vi "Function_Find Circle #2.vi"(7 "功能":enum16{"半徑", "毛邊"}(ring), 8 "Error in":errorcluster, 9 "CoordSys In":T2 {"Measurement System"."Axis Reference" items=["Direct", "Indirect"]; "Measurement System"."Angle (deg)" format="%.2f"; "Measurement System"."Origin"."Y" format="%.2f"; "Measurement System"."Origin"."X" format="%.2f"; "Reference System"."Axis Reference" items=["Direct", "Indirect"]; "Reference System"."Angle (deg)" format="%.2f"; "Reference System"."Origin"."Y" format="%.2f"; "Reference System"."Origin"."X" format="%.2f"}, 10 "Data Cluster In":cluster{"Name":string, "Variant In":variant}, 11 "Image Src":T4) -> (0 "Error Out":errorcluster, 1 "Max & min":T1 {"Min Position"."Y" format="%.2f"; "Min Position"."X" format="%.2f"; "Max Position"."Y" format="%.2f"; "Max Position"."X" format="%.2f"}, 2 "Result(Circ)":cluster{"Name":string, "NG?":bool, "Score":dbl}, 3 "Result":T3 {"Center"."Y" format="%.2f"; "Center"."X" format="%.2f"}, 4 "Time":u32)   [LabVIEW 2013]
uses:
  <vilib>/vision/Image Controls.llb/IMAQ Image.ctl
  Control/Control Find Circle #2.ctl
  <vilib>/vision/Measure.llb/Edge Options.ctl
  <vilib>/vision/Measure.llb/Edge Polarity.ctl
  <vilib>/vision/NI_Vision_Development_Module.lvlib
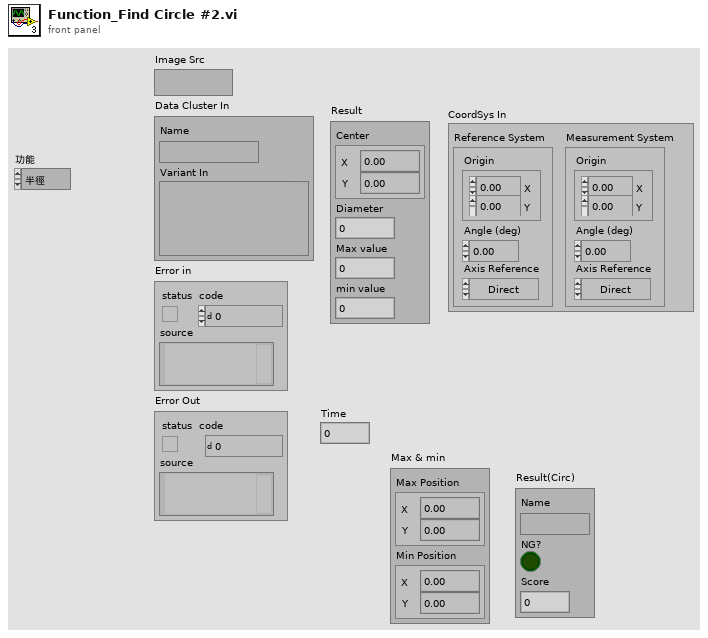
[diagram p1: front panel]
types:
  T1 = cluster{"Max Position":cluster{"X":sgl, "Y":sgl}, "Min Position":cluster{"X":sgl, "Y":sgl}}
  T2 = typedef "IMAQ Coordinate System" = cluster{"Reference System":cluster{"Origin":cluster{"X":sgl, "Y":sgl}, "Angle (deg)":sgl, "Axis Reference":u32}, "Measurement System":cluster{"Origin":cluster{"X":sgl, "Y":sgl}, "Angle (deg)":sgl, "Axis Reference":u32}}
  T3 = cluster{"Center":cluster{"X":sgl, "Y":sgl}, "Diameter":dbl, "Max value":sgl, "min value":sgl}
  T4 = typedef "IMAQ Image.ctl" = refnum<image>
  T5 = typedef "Control Find Circle #2.ctl" = cluster{"ROI Descriptor":cluster{"Global Rectangle":i32[], "Contours":cluster{"ID":enum32{"External", "Internal"}, "Type":u32, "Coordinates":i32[]}[]}, "Edge Options":cluster{"Edge Options":T6, "Step Size":dbl, "Scan Direction":u16, "Auto":bool, "SD":dbl}, "條件":cluster{"半徑最大值":dbl, "半徑最小值":dbl}}
  T6 = typedef "Edge Options.ctl" = cluster{"Edge Polarity":T7, "Kernel Size":u32, "Width":u32, "Minimum Edge Strength":sgl, "Interpolation Type":enum32{"Zero Order", "Bilinear", "Quadratic", "Cubic", "Bilinear Fixed"}, "Data Processing Method":enum32{"Average", "Median"}}
  T7 = typedef "Edge Polarity.ctl" = u32
  T8 = cluster{"Center":cluster{"X":sgl, "Y":sgl}, "Radius":dbl, "Max value":sgl, "min value":sgl}
  T9 = cluster{"Global Rectangle":i32[], "Contours":cluster{"ID":enum32{"External", "Internal"}, "Type":u32, "Coordinates":i32[]}[]}
  T10 = cluster{"Origin":cluster{"X":sgl, "Y":sgl}, "Angle (deg)":sgl, "Axis Reference":u32}
  T11 = typedef "ROI Descriptor" = cluster{"Global Rectangle":i32[], "Contours":cluster{"ID":enum32{"External", "Internal"}, "Type":u32, "Coordinates":i32[]}[]}
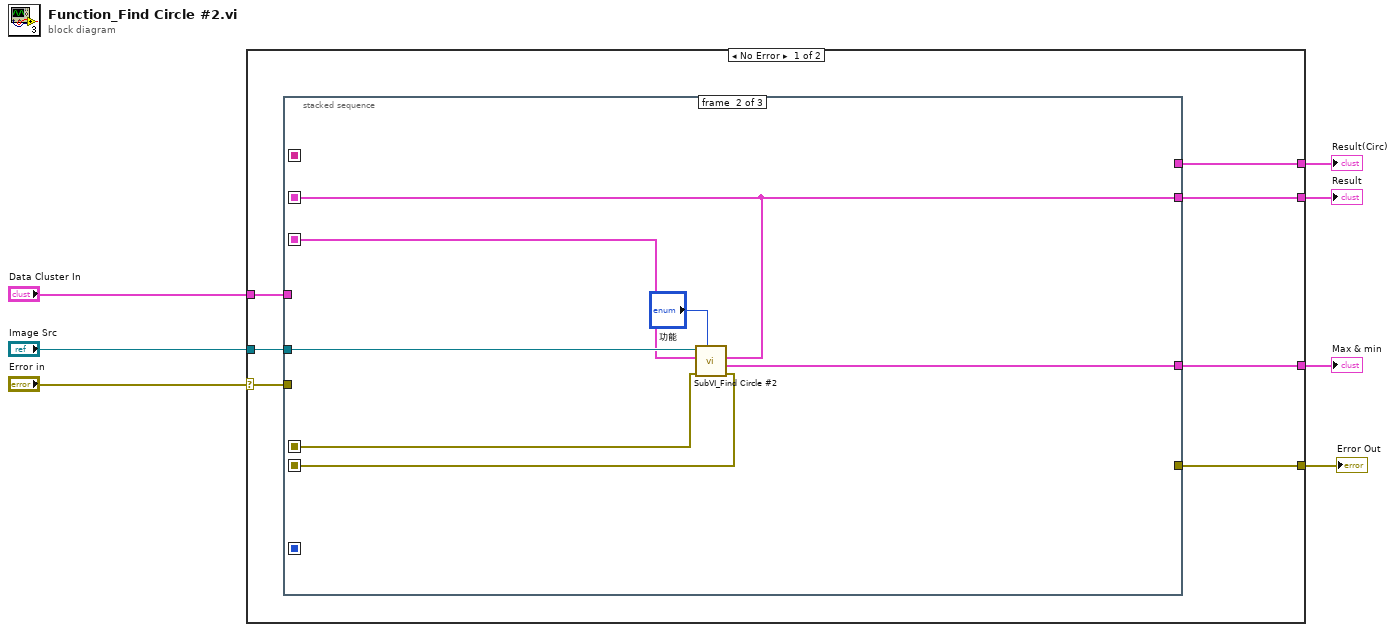
[diagram p0: block diagram]
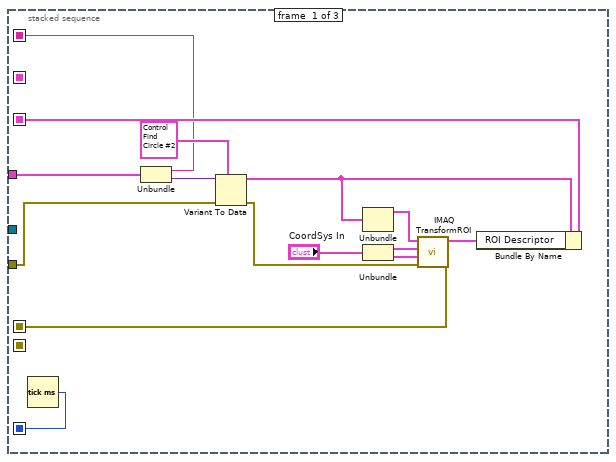
[diagram p2: hidden frame]
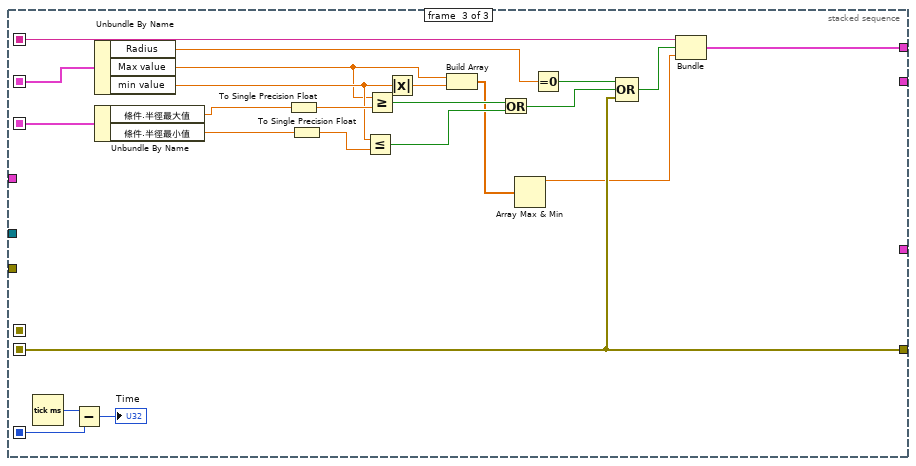
[diagram p3: hidden frame]
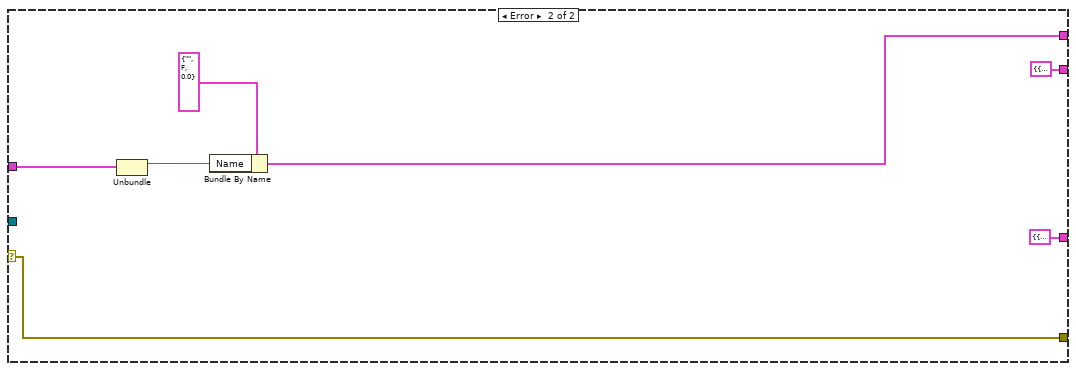
[diagram p4: hidden frame]
diagram:
  n1 = case shown="No Error" "Error in" {
    selector: "Error in" -> [w8 w64]
    tunnel: "Image Src" -> [w14 _]
    tunnel: "Data Cluster In" -> [w13 w63]
    tunnel: [w12 w61] -> w5
    tunnel: [w11 T8 {"Center"={"X"=0.0, "Y"=0.0}, "Radius"=0.0, "Max value"=0.0, "min value"=0.0} ("Result_Circle")] -> w4
    tunnel: [w10 T1 {"Max Position"={"X"=0.0, "Y"=0.0}, "Min Position"={"X"=0.0, "Y"=0.0}} ("Max & min")] -> w3
    tunnel: [w9 w64] -> w1
    frame No Error {
      n2 = stacked-sequence {
        seq-local: [w24 _ _] -> [_ w35 w50]
        seq-local: [w20 _ _] -> [_ _ w58]
        seq-local: [w19 _ _] -> [_ _ w53]
        seq-local: [_ w32 _] -> [_ _ w54]
        seq-local: [_ w34 _] -> [_ _ w51]
        seq-local: [w18 _ _] -> [_ w33 _]
        tunnel: w8 -> [w17 _ _]
        tunnel: w14 -> [_ w36 _]
        tunnel: [_ _ w51] -> w9
        tunnel: [_ _ w52] -> w12
        tunnel: w13 -> [w15 _ _]
        tunnel: [_ w32 _] -> w11
        tunnel: [_ w31 _] -> w10
        frame #0 {
          n3 = Tick Count (ms)() -> (millisecond timer value=w20:u32)
          n4 = Unbundle(w15) -> ("Name"=w19:string, "Variant In"=w29:variant)
          n5 = Variant To Data(error in=w17, type=T5 {"ROI Descriptor"={"Global Rectangle"=[], "Contours"=[]}, "Edge Options"={"Edge Options"={"Edge Polarity"=0, "Kernel Size"=0, "Width"=0, "Minimum Edge Strength"=0.0, "Interpolation Type"=enum."Zero Order", "Data Processing Method"=enum."Average"}, "Step Size"=3.0, "Scan Direction"=0, "Auto"=FALSE, "SD"=0.0}, "條件"={"半徑最大值"=0.0, "半徑最小值"=0.0}} ("Parameter_Circle"), Variant=w29) -> (data=w22:T5, error out=w16:errorcluster)
          n6 = Unbundle(w22) -> ("ROI Descriptor"=w21:T9)  [unwired: 2 out]
          n7 = Unbundle("CoordSys In") -> ("Reference System"=w26:T10, "Measurement System"=w27:T10)
          n8 = call "IMAQ TransformROI"("error in (no error)"=w16, "New Reference"=w27, "Base Reference"=w26, "ROI Descriptor"=w21) -> ("error out"=w18:errorcluster, "ROI Descriptor out"=w23:T11)  [unwired: 6 in]
          n9 = Bundle By Name(cluster=w22, "ROI Descriptor"=w23) -> (w24:T5)
        }
        frame #1 {
          n10 = call "SubVI_Find Circle #2.vi"("功能"="功能", "error in"=w33, "Parameter_Circle"=w35, "Image in"=w36) -> ("error out"=w34:errorcluster, "Max & min"=w31:T1, "Result_Circle"=w32:T8)  [unwired: 4 in, 1 out]
        }
        frame #2 {
          n11 = Tick Count (ms)() -> (millisecond timer value=w59:u32)
          n12 = Subtract(x=w59, y=w58) -> (x-y=→"Time":u32)
          n13 = Unbundle By Name(w54) -> ("Radius"=w42:dbl, "Max value"=w39:sgl, "min value"=w41:sgl)
          n14 = Unbundle By Name(w50) -> ("條件.半徑最大值"=w49:dbl, "條件.半徑最小值"=w48:dbl)
          n15 = To Single Precision Float(number=w49) -> (single precision float=w47:sgl)
          n16 = To Single Precision Float(number=w48) -> (single precision float=w46:sgl)
          n17 = Less Or Equal?(x=w41, y=w46) -> (x <= y?=w44:bool)
          n18 = Greater Or Equal?(x=w39, y=w47) -> (x >= y?=w45:bool)
          n19 = Absolute Value(x=w41) -> (abs(x)=w40:sgl)
          n20 = Build Array(w39, w40) -> (w38:sgl[])
          n21 = Or(x=w45, y=w44) -> (x .or. y?=w43:bool)
          n22 = Array Max & Min(array=w38) -> (max value=w37:sgl)  [unwired: 3 out]
          n23 = Equal To 0?(x=w42) -> (x = 0?=w55:bool)
          n24 = Compound Arithmetic op=OR(w55, w43, w51) -> (w56:bool)
          n25 = Bundle("Name"=w53, w56, w37) -> (w52:cluster{"Name":string, bool, sgl})  [unwired: 1 in]
        }
      }
    }
    frame Error {
      n26 = Unbundle(w63) -> ("Name"=w60:string)  [unwired: 1 out]
      n27 = Bundle By Name(cluster=cluster{"Name":string, bool, "Radius":dbl} {"Name"="", FALSE, "Radius"=0.0}, "Name"=w60) -> (w61:cluster{"Name":string, bool, "Radius":dbl})
    }
  }
  "Result(Circ)" <- w5
  "Result" <- w4
  "Max & min" <- w3
  "Error Out" <- w1
